vi "ArrayOfPathComponentStrings.vi"(1 "PathStringIn":string) -> (0 "ArrayOfPathComponentStringsOut":string[](array[string]))   [LabVIEW 2022 SP3]
panel:
  out "array of strings":string[](array[string])
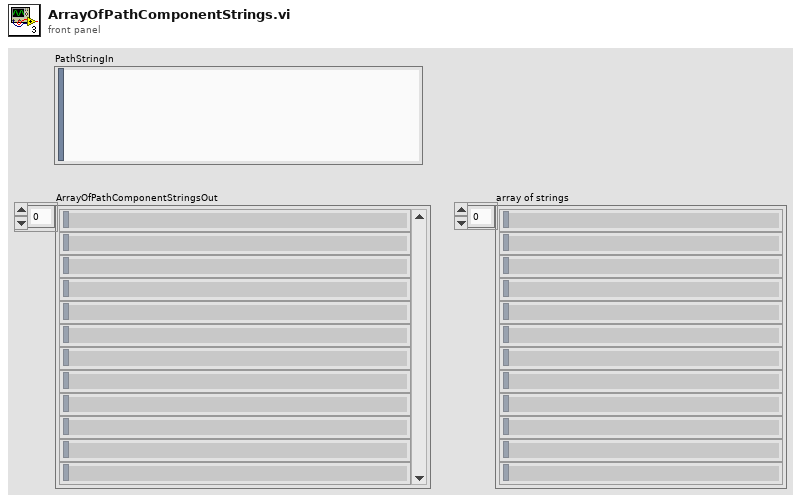
[diagram p1: front panel]
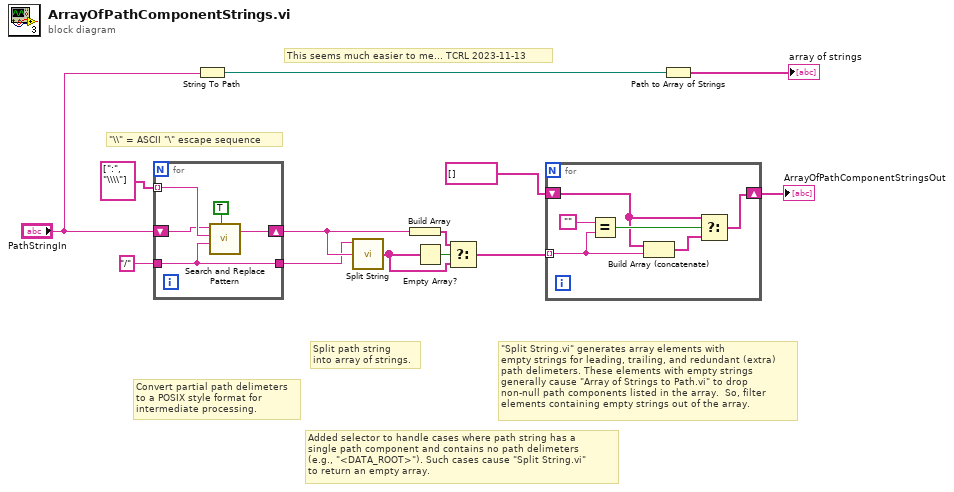
[diagram p0: block diagram]
diagram:
  # "This seems much easier to me... TCRL 2023-11-13"
  # "Added selector to handle cases where path string has a \nsingle path component and contains no path delimeters\n(e.g., \"<DATA_ROOT>\"). Such cases cause \"Split String.vi\"\nto return an empty array."
  # "\"Split String.vi\" generates array elements with\nempty strings for leading, trailing, and redundant (extra)\npath delimeters. These elements with empty strings \ngenerally cause \"Array of Strings to Path.vi\" to drop \nnon-null path components listed in the array.  So, filter\nelements containing empty strings out of the array."
  # "Split path string\ninto array of strings."
  # "Convert partial path delimeters\nto a POSIX style format for\nintermediate processing."
  # "\"\\\\\" = ASCII \"\\\" escape sequence"
  n1 = for {
    tunnel: string[] [":", "\\\\"] -> [w18] mode=indexing
    shift-right: [w16] -> w12
    shift-left: "PathStringIn" -> [w15]
    tunnel: "/" ("replace string (\"\")") -> [w14]
    tunnel: [w14] -> w4
    n2 = call <vilib>:"Search and Replace Pattern.vi"("string"=w15, "regular expression (\"\")"=w18, "replace string (\"\")"=w14, "replace all? (F)"=TRUE) -> ("result string"=w16:string)  [unwired: 1 in, 1 out]
  }
  n3 = String To Path(string="PathStringIn") -> (path=w2:path)
  n4 = call <vilib>:"Split String.vi"("Split Pattern"=w4, "Input String"=w12) -> ("Split String"=w10:string[])  [unwired: 5 in]
  n5 = Build Array(w12) -> (w11:string[])
  n6 = Empty Array?(array=w10) -> (empty?=w9:bool)
  n7 = Select(t=w11, s=w9, f=w10) -> (s? t:f=w13:string[])
  n8 = for {
    shift-right: [w22] -> w5
    shift-left: string[] [] -> [w21]
    tunnel: w13 -> [w20] mode=indexing
    n9 = Equal?(x="", y=w20) -> (x = y?=w23:bool)
    n10 = Build Array (concatenate)(w21, w20) -> (w19:string[])
    n11 = Select(t=w21, s=w23, f=w19) -> (s? t:f=w22:string[])
  }
  "ArrayOfPathComponentStringsOut" <- w5
  n12 = Path to Array of Strings(0:w2) -> (2:→"array of strings":string[])  [unwired: 1 out]
